vi "Pre Launch Init.vi"(11 "Guardian in":refnum<class "Guardian.lvclass">) -> (0 "error out":errorcluster, 3 "Guardian out":refnum<class "Guardian.lvclass">)   [LabVIEW 2026, in "TALOS.lvlib" / "Guardian.lvlib" / "Guardian.lvclass"]
doc: "(<B>Filename</B>: Actor Framework.lvlib:Actor.lvclass:Pre Launch Init.vi)\n\nDefines behavior that occurs after the Launch Nested Actor method is invoked but before the actor's Actor Core method begins running.\n\nBy default, this method does nothing. A descendant class may override it to define behavior."
uses:
  Guardian.lvclass
  Guardian.lvclass/Guardian.ctl
  Ancestor/Ancestor/Ancestor.lvclass/Ancestor.ctl
  Support VIs/Substitute Error.vi
  Support VIs/Generate Error.vi
  FGV/Error Memory/Get Error Description.vi
  Support VIs/Get PC name.vi
  Ancestor/Ancestor/Read ID.vi
  Support VIs/Get Class Name.vi
  <vilib>/Utility/error.llb/Clear Errors.vi
  FGV/Error Memory/Error Memory Core.vi
  <vilib>/AdvancedString/Delimited String to 1D String Array.vi
  <vilib>/AdvancedString/Delimited String to 1D String Array (string).vi
  Support VIs/Circus Root Path.vi
  FGV/Error Memory/Error Crt Lvl checker.vi
  FGV/Error Memory/Error Memory Core.vi/40c8088d-b597-4017-91af-faa98e00292e.vi
  FGV/Error Memory/Error Memory Core.vi/d4a3ab98-063c-4e44-b43d-fbdcfe6c2be2.vi
  Support VIs/Global Memory.vi
  <vilib>/Utility/LVClass/Get LV Class Name.vi
  Support VIs/Is in Packed Library.vi
  Support VIs/TALOS Root path.vi
  Support VIs/Read CSV worksheet.vi
  Support VIs/Global Constants.vi
  <vilib>/Utility/error.llb/General Error Handler.vi
  Support VIs/Error Log.vi
  Ancestor/Ancestor/Ancestor.lvclass
  <vilib>/Comparison/Equal/Equal Functor/Equal Functor.lvclass
  TALOS.lvlib
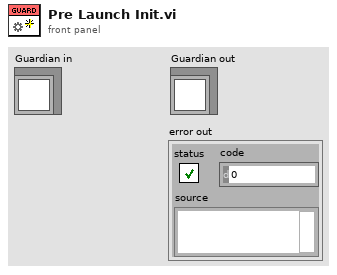
[diagram p1: front panel]
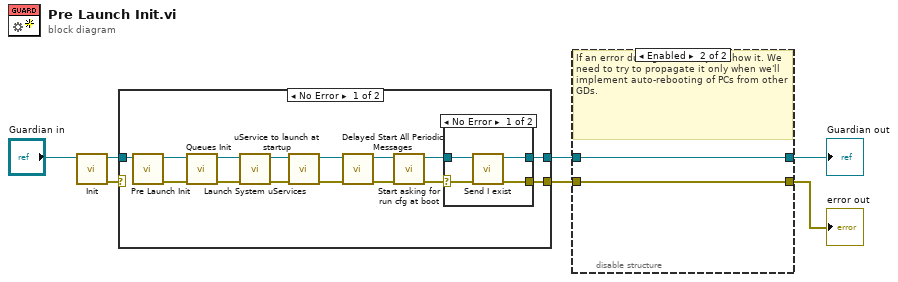
[diagram p0: block diagram]
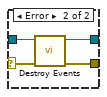
[diagram p2: hidden frame]
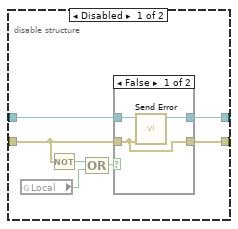
[diagram p4: hidden frame]
diagram:
  n1 = call "Init.vi"("Guardian in"="Guardian in") -> ("error out"=w5:errorcluster, "Guardian out"=w7:refnum<class "Guardian.lvclass">)  [unwired: 9 in]
  n2 = case shown="No Error" w5 {
    selector: w5 -> [_ w31]
    tunnel: [w19 w32] -> w4
    tunnel: [w18 w31] -> w1
    tunnel: w7 -> [w20 w32]
    frame No Error {
      n3 = call-parent "Pre Launch Init.vi"("Ancestor in"=w20) -> ("error out"=w21:errorcluster, "Ancestor out"=w22:refnum<class "Guardian.lvclass">)  [unwired: 9 in]
      n4 = call "Queues Init.vi"("error in (no error)"=w21, "Guardian in"=w22) -> ("error out"=w14:errorcluster, "Guardian out"=w15:refnum<class "Guardian.lvclass">)  [unwired: 8 in]
      n5 = call "Launch System uServices.vi"("error in (no error)"=w14, "Guardian in"=w15) -> ("error out"=w16:errorcluster, "Guardian out"=w17:refnum<class "Guardian.lvclass">)  [unwired: 8 in]
      n6 = call "uService to launch at startup.vi"("error in (no error)"=w16, "Guardian in"=w17) -> ("error out"=w12:errorcluster, "Guardian out"=w13:refnum<class "Guardian.lvclass">)  [unwired: 8 in]
      n7 = call "Delayed Start All Periodic Messages.vi"("error in (no error)"=w12, "Guardian in"=w13) -> ("error out"=w11:errorcluster, "Guardian out"=w9:refnum<class "Guardian.lvclass">)  [unwired: 8 in]
      n8 = call-dynamic "Start asking for run cfg at boot.vi"("error in (no error)"=w11, "Guardian in"=w9) -> ("error out"=w10:errorcluster, "Guardian out"=w8:refnum<class "Guardian.lvclass">)  [unwired: 8 in]
      n9 = case shown="No Error" w10 {
        selector: w10 -> [w24 w28]
        tunnel: w8 -> [w26 w30]
        tunnel: [w25 w29] -> w19
        tunnel: [w23 w27] -> w18
        frame No Error {
          n10 = call "Send I exist.vi"("error in (no error)"=w24, "Guardian in"=w26) -> ("error out"=w23:errorcluster, "Guardian out"=w25:refnum<class "Guardian.lvclass">)  [unwired: 8 in]
        }
        frame Error {
          n11 = call-dynamic "Destroy Events.vi"("error in (no error)"=w28, "Guardian in"=w30) -> ("error out"=w27:errorcluster, "Guardian out"=w29:refnum<class "Guardian.lvclass">)  [unwired: 8 in]
        }
      }
    }
    frame Error {
    }
  }
  n12 = disable-structure shown="Enabled" {
    disable-tunnel: w4 -> [w39 w46]
    disable-tunnel: [w38 w46] -> w3
    disable-tunnel: [w37 w45] -> w2
    disable-tunnel: w1 -> [w35 w45]
    frame Disabled {
      n13 = global read "Global Constants.vi" "Local"() -> (w34:bool)
      n14 = Not(x=w35) -> (.not. x?=w33:bool)
      n15 = Compound Arithmetic op=OR(w33, w34) -> (w36:bool)
      n16 = case shown="False" w36 {
        tunnel: w39 -> [w42 w44]
        tunnel: [w41 w44] -> w38
        tunnel: [w40 w43] -> w37
        tunnel: w35 -> [w40 w43]
        frame False {
          n17 = call-dynamic "Send Error.vi"("error in (no error)"=w40, "Guardian in"=w42) -> ("Guardian out"=w41:refnum<class "Guardian.lvclass">)  [unwired: 8 in, 1 out]
        }
        frame True {
        }
      }
    }
    frame Enabled {
      # "If an error during Init, let's just show it. We need to try to propagate it only when we'll implement auto-rebooting of PCs from other GDs."
    }
  }
  "error out" <- w2
  "Guardian out" <- w3
